vi "Help.vi"(8 "error In":errorcluster) -> (0 "error Out":errorcluster)   [LabVIEW 2014]
panel:
  # "Exercise Help"
  # "Preenchimento dos campos\n\nTolerância da Resposta\n\nDados são salvos a cada vez que se sai do enunciado\n\nem caso de erros inesperados o que fazer?"
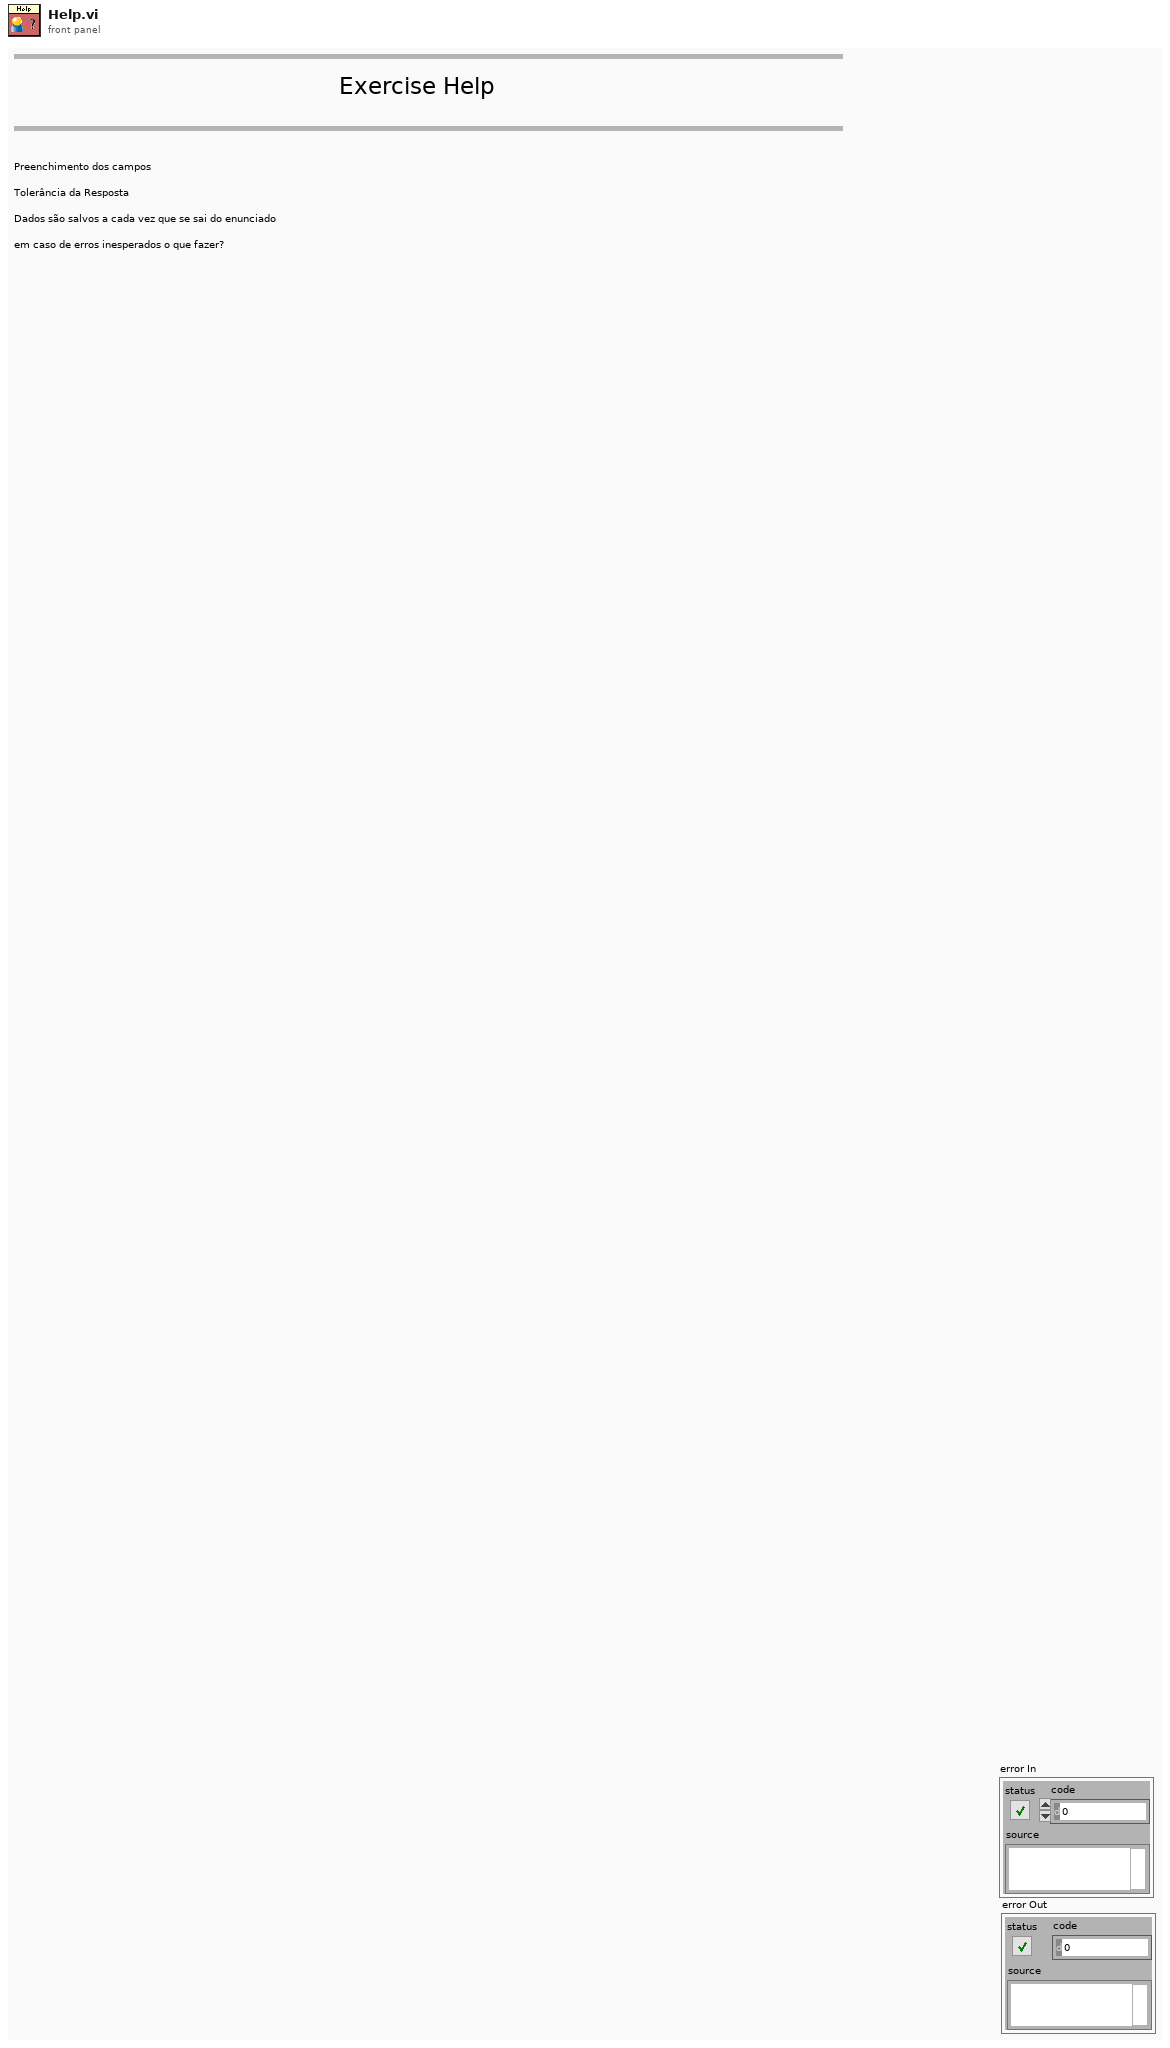
[diagram p1: front panel]
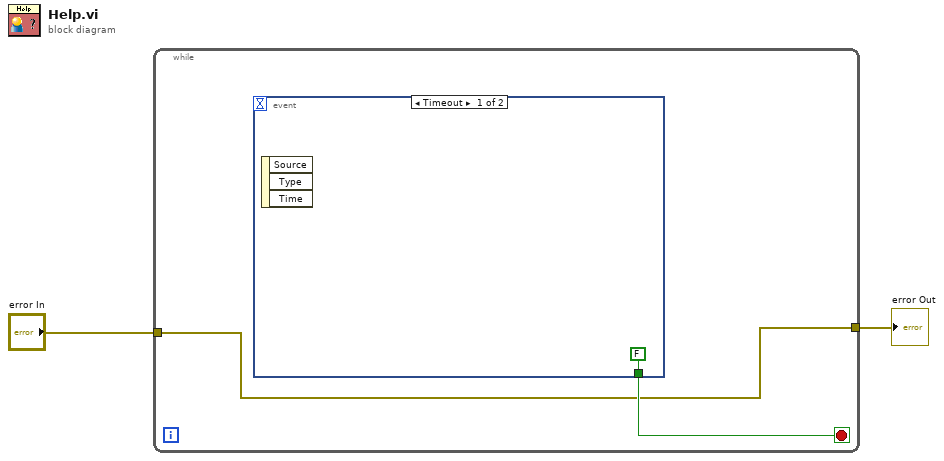
[diagram p0: block diagram]
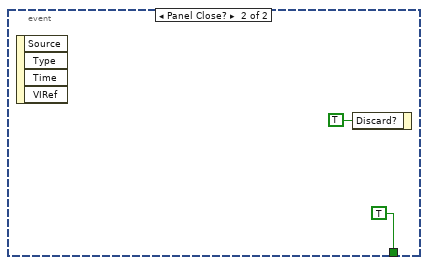
[diagram p2: hidden frame]
diagram:
  n1 = while {
    tunnel: "error In" -> [w3]
    tunnel: [w3] -> w1
    stop <- w4 stop-if-true
    n2 = event shown="[0] Timeout" {
      selector: _ -> [_ _]
      dyn-events: _ -> [_ _]
      timeout: _ -> [_ _]
      tunnel: [FALSE TRUE] -> w4
      event Timeout {
        n3 = event-data() -> ()  [unwired: 1 in, 3 out]
      }
      event Panel Close? {
        n4 = event-data() -> ()  [unwired: 1 in, 4 out]
        n5 = event-data("Discard?"=TRUE) -> ()  [unwired: 1 in, 1 out]
      }
    }
  }
  "error Out" <- w1
